vi "DO sat.vi"(10 "Atmospheric Pressure (kPa)":dbl format="%.2f", 11 "Temperature (C)":dbl format="%.2f") -> (3 "DO sat (mg/L)":dbl format="%.2f")   [LabVIEW 2012]
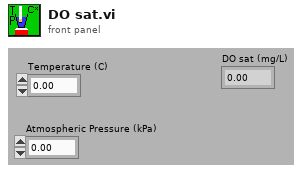
[diagram p1: front panel]
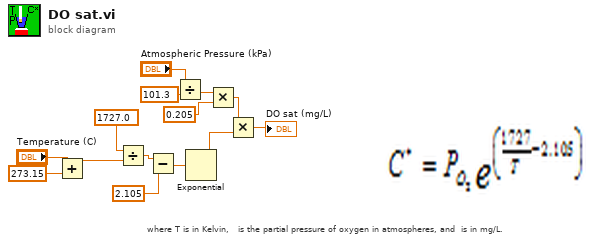
[diagram p0: block diagram]
diagram:
  # "where T is in Kelvin,   is the partial pressure of oxygen in atmospheres, and  is in mg/L."
  n1 = Add(x="Temperature (C)", y=273.15) -> (x+y=w7:dbl)
  n2 = Divide(x=1727.0 ("y"), y=w7) -> (x/y=w6:dbl)
  n3 = Subtract(x=w6, y=2.105) -> (x-y=w4:dbl)
  n4 = Divide(x="Atmospheric Pressure (kPa)", y=101.3) -> (x/y=w10:dbl)
  n5 = Exponential(1:w4) -> (0:w3:dbl)
  n6 = Multiply(x=w10, y=0.205) -> (x*y=w2:dbl)
  n7 = Multiply(x=w2, y=w3) -> (x*y=→"DO sat (mg/L)":dbl)
